vi "Pointer Test.vi"() -> ()   [LabVIEW 2019]
uses:
  <vilib>/gpm_packages/@cs/linked-list/Source/Linked List/Linked List/Linked List.lvclass
  C:/Program Files/National Instruments/LabVIEW 2019/vi.lib/gpm_packages/@cs/linked-list/Source/Linked List/ILinkedList/ILinked List.lvclass
  85e8f493-8fd8-44fa-aed1-18b72ad78bbc.vi
  a7220b0b-566b-4baf-a18c-d3612f3f69c2.vi
  40ee21ff-095a-4008-8703-87659f5f828c.vi
  1be2ee1e-190a-4265-9413-3625170d492e.vi
  63f81286-0c53-4584-b61d-bde98da1fb55.vi
  d0ecef96-780f-4e76-ac67-b51bdb239ee9.vi
  <vilib>/gpm_packages/@cs/linked-list/Source/Linked List/ILinkedList/ILinked List.lvclass
  <vilib>/gpm_packages/@cs/linked-list/Source/Linked List/Linked List Ref/Linked List Ref.lvclass
panel:
  in  "Tree 2":string(tree)
  out "error out":errorcluster
  out "Pointer Attribute Name":string
  out "Pointer?":bool
  out "Pointer ID":string
  out "Data ID":string
  out "Attribute Name out":string
  out "Attribute":i32
  in  "Tree":string(tree)
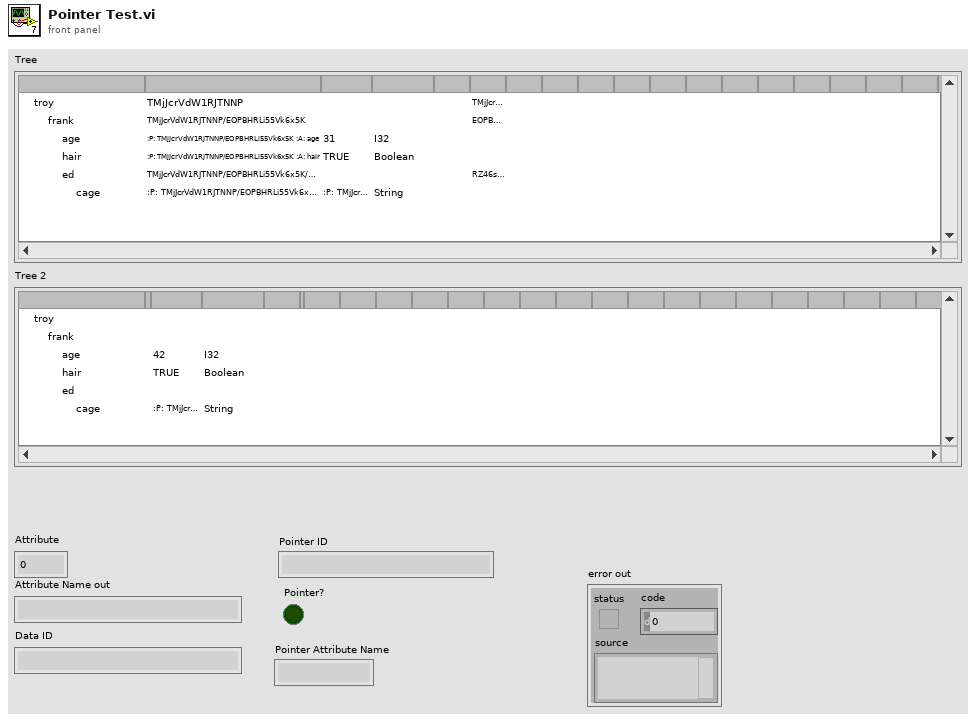
[diagram p1: front panel]
types:
  T1 = cluster{"Left Cell String":string, "Child Text":string[], "Child Tag":string, "Item Indent":i32, "Child Only?":bool, "Glyph Index":i32}[]
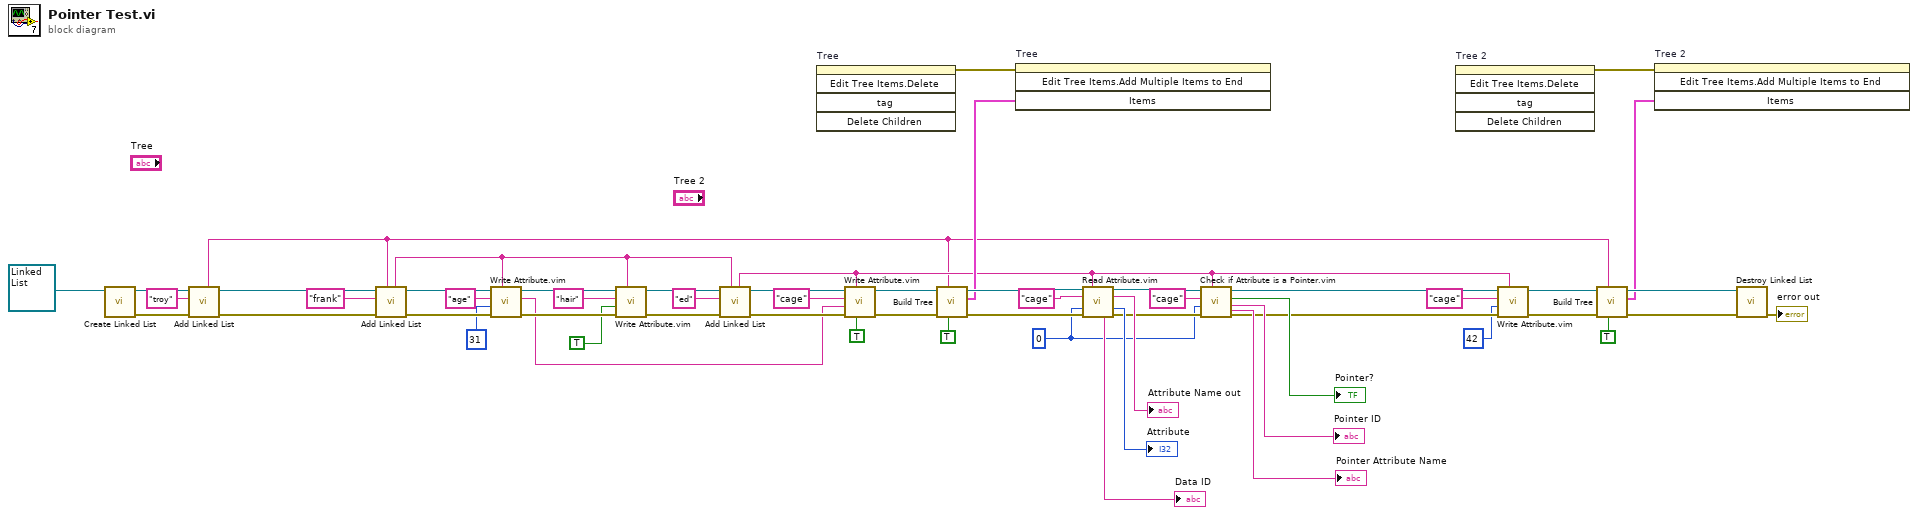
[diagram p0: block diagram]
diagram:
  w16 = 0
  n1 = call <vilib>:"Create Linked List.vi"("Linked List"=refnum<class "Linked List.lvclass"> refnum ("Dictionary.lvlib:Dictionary.lvclass")) -> ("error out"=w44:errorcluster, "Linked List Ref"=w46:refnum<data-value>)  [unwired: 9 in]
  n2 = call <vilib>:"Add Linked List.vi"("error in (no error)"=w44, "Name"="troy" ("Dictionary Name"), "Linked List Ref"=w46) -> ("error out"=w43:errorcluster, "Linked List Ref out"=w45:refnum<data-value>, "Linked List ID out"=w3:string)  [unwired: 5 in, 1 out]
  n3 = call <vilib>:"Add Linked List.vi"("Parent ID"=w3, "error in (no error)"=w43, "Name"="frank", "Linked List Ref"=w45) -> ("error out"=w53:errorcluster, "Linked List Ref out"=w54:refnum<data-value>, "Linked List ID out"=w37:string)  [unwired: 4 in, 1 out]
  n4 = call "Write Attribute.vim"("Linked List ID"=w37, "error in (no error)"=w53, "Attribute"=31, "Attribute Name"="age", "Linked List Ref"=w54) -> ("error out"=w49:errorcluster, "Attribute ID out"=w33:string, "Linked List Ref out"=w50:refnum<data-value>)  [unwired: 3 in, 1 out]
  n5 = call "Write Attribute.vim"("Linked List ID"=w37, "error in (no error)"=w49, "Attribute"=TRUE, "Attribute Name"="hair", "Linked List Ref"=w50) -> ("error out"=w35:errorcluster, "Linked List Ref out"=w36:refnum<data-value>)  [unwired: 3 in, 2 out]
  n6 = call <vilib>:"Add Linked List.vi"("Parent ID"=w37, "error in (no error)"=w35, "Name"="ed", "Linked List Ref"=w36) -> ("error out"=w38:errorcluster, "Linked List Ref out"=w39:refnum<data-value>, "Linked List ID out"=w9:string)  [unwired: 4 in, 1 out]
  n7 = invoke on="Tree" class="Tree (strict)" method="Edit Tree Items.Delete"() -> (error out=w41:errorcluster)  [unwired: 5 in, 4 out]
  n8 = call "Write Attribute.vim"("Pointer?"=TRUE, "Linked List ID"=w9, "error in (no error)"=w38, "Attribute"=w33, "Attribute Name"="cage", "Linked List Ref"=w39) -> ("error out"=w28:errorcluster, "Linked List Ref out"=w30:refnum<data-value>)  [unwired: 2 in, 2 out]
  n9 = call <vilib>:"Build Tree.vi"("Show IDs"=TRUE, "Linked List ID"=w3, "error in (no error)"=w28, "Linked List Ref"=w30) -> ("error out"=w27:errorcluster, "Tree Data"=w26:T1, "Linked List Ref out"=w29:refnum<data-value>)  [unwired: 5 in]
  n10 = invoke on="Tree" class="Tree (strict)" method="Edit Tree Items.Add Multiple Items to End"(error in=w41, "Items"=w26) -> ()  [unwired: 2 in, 4 out]
  n11 = call "Read Attribute.vim"("Linked List Ref"=w29, "Linked List ID"=w9, "Attribute Name"="cage", "Type"=w16, "error in (no error)"=w27) -> ("Linked List Ref out"=w21:refnum<data-value>, "Attribute Name out"=→"Attribute Name out":string, "Attribute"=→"Attribute":i32, "Data ID"=→"Data ID":string, "error out"=w20:errorcluster)  [unwired: 5 in, 1 out]
  n12 = call "Check if Attribute is a Pointer.vim"("Linked List ID"=w9, "error in (no error)"=w20, "Type"=w16, "Attribute Name"="cage", "Linked List Ref"=w21) -> ("error out"=w11:errorcluster, "Pointer ID"=→"Pointer ID":string, "Pointer?"=→"Pointer?":bool, "Linked List Ref out"=w12:refnum<data-value>, "Pointer Attribute Name"=→"Pointer Attribute Name":string)  [unwired: 2 in]
  n13 = invoke on="Tree 2" class="Tree (strict)" method="Edit Tree Items.Delete"() -> (error out=w2:errorcluster)  [unwired: 5 in, 4 out]
  n14 = call "Write Attribute.vim"("Linked List ID"=w9, "error in (no error)"=w11, "Attribute"=42, "Attribute Name"="cage", "Linked List Ref"=w12) -> ("error out"=w5:errorcluster, "Linked List Ref out"=w7:refnum<data-value>)  [unwired: 3 in, 2 out]
  n15 = call <vilib>:"Build Tree.vi"("Show IDs"=TRUE, "Linked List ID"=w3, "error in (no error)"=w5, "Linked List Ref"=w7) -> ("error out"=w4:errorcluster, "Tree Data"=w1:T1, "Linked List Ref out"=w6:refnum<data-value>)  [unwired: 5 in]
  n16 = invoke on="Tree 2" class="Tree (strict)" method="Edit Tree Items.Add Multiple Items to End"(error in=w2, "Items"=w1) -> ()  [unwired: 2 in, 4 out]
  n17 = call <vilib>:"Destroy Linked List.vi"("error in (no error)"=w4, "Linked List Ref"=w6) -> ("error out"=→"error out":errorcluster)  [unwired: 9 in]
